vi "VsEP Init Data File.vi"(0 "Expt State":T5, 1 "Params":T2 {"STIMULUS"."dB STEPSIZE" format="%#_3g"; "STIMULUS"."START dB re 1g/ms" step=5}, 7 "Max Jerk (dB re 1 g/ms)":dbl, 11 "error in (no error)":errorcluster) -> (4 "Expt State out":T5, 6 "Datafile path":path, 15 "error out":errorcluster)   [LabVIEW 2020]
uses:
  CFTS Main Panel SubVIs/CFTS-Experiment State.ctl
  Typedefs/VsEP-Parameters.ctl
  Typedefs/VsEP-Stimulus Control.ctl
  Typedefs/VsEP-Hidden Params.ctl
  epl-vi-lib/Signal Synthesis VIs/Controls/Gate XCtl/Gate Control.xctl
  CFTS Main Panel SubVIs/CFTS-Data Type Enum.ctl
  epl-vi-lib/Utility VIs/File IO VIs/Configuration File Wrapper VIs/Config-Read Key (string).vi
panel:
  in  "VsEP Data File":T1
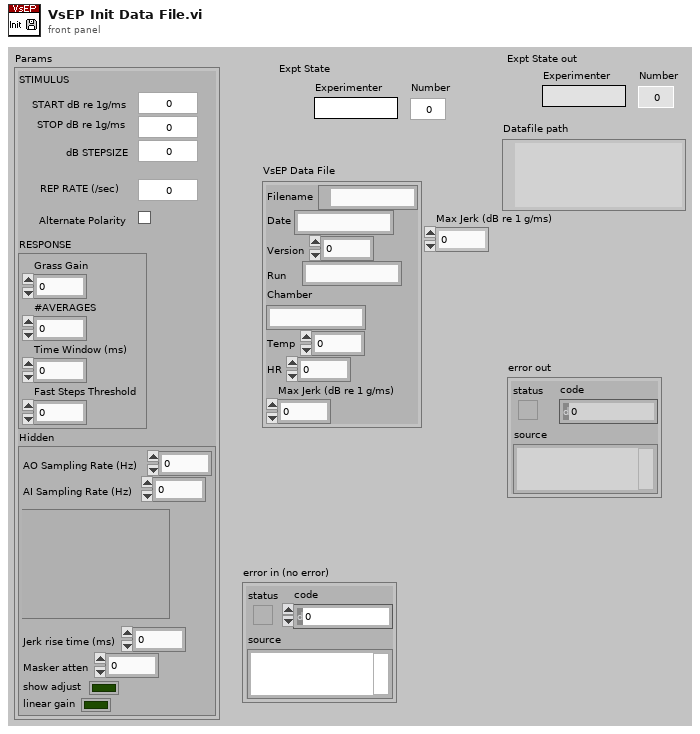
[diagram p1: front panel]
types:
  T1 = cluster{"Filename":path, "Date":string, "Version":i32, "Run":string, "Chamber":string, "Temp":dbl, "HR":dbl, "Max Jerk (dB re 1 g/ms)":dbl}
  T2 = typedef "VsEP-Parameters.ctl" = cluster{"STIMULUS":T3, "RESPONSE":cluster{"Grass Gain":i32, "#AVERAGES":i32, "Time Window (ms)":sgl, "Fast Steps Threshold":i32}, "Hidden":T4}
  T3 = typedef "VsEP-Stimulus Control.ctl" = cluster{"START dB re 1g/ms":i32, "STOP dB re 1g/ms":i32, "dB STEPSIZE":sgl, "REP RATE (/sec)":dbl, "Alternate Polarity":bool, "Sampling Rate (Hz)":dbl}
  T4 = typedef "VsEP-Hidden Params.ctl" = cluster{"AO Sampling Rate (Hz)":dbl, "AI Sampling Rate (Hz)":dbl, "Masker Timing":cluster{"Active":bool, "Delay (ms)":dbl, "Width (ms)":dbl, "Ramp (ms)":dbl}, "Jerk rise time (ms)":dbl, "Masker atten":dbl, "show adjust":bool, "linear gain":bool}
  T5 = typedef "CFTS-Experiment State.ctl" = cluster{"Experimenter":string, "Number":u32, "Right":string, "Left":string, "Data Folder":path, "State File":path, "Version Info":string, "End Exposure Time":dbl, "Exposure Duration":string, "Run #":cluster{"CAP":i16, "ABR":i16, "DP":i16, "VsEP":i16, "MeasSeq":i16, "SubSeq":i16, "SFOAE":i16}}
  T6 = typedef "CFTS-Data Type Enum.ctl" = enum16{"CAP", "ABR", "DP", "VsEP", "MeasSeq", "SFOAE"}
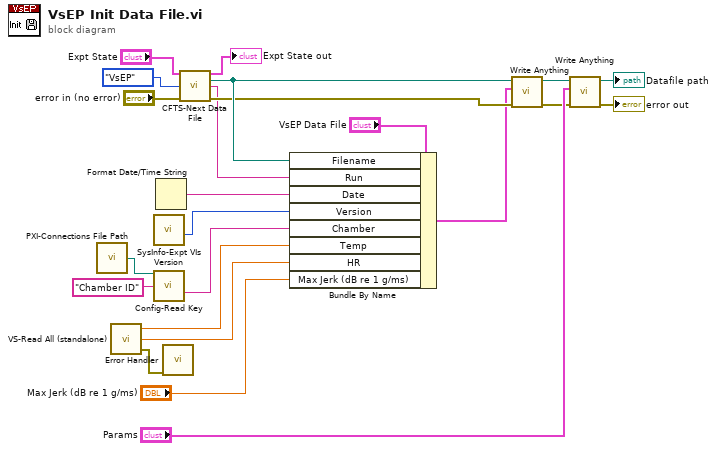
[diagram p0: block diagram]
diagram:
  n1 = call "PXI-Connections File Path.vi"() -> ("Path"=w17:path)  [unwired: 1 in]
  n2 = call "VS-Read All (standalone).vi"() -> ("error out"=w19:errorcluster, "Heart Rate (bpm)"=w3:dbl, "Temperature (C)"=w4:dbl)  [unwired: 3 in]
  n3 = call "SysInfo-Expt VIs Version.vi"() -> ("Expt VIs Version out"=w10:i32)  [unwired: 11 in]
  n4 = call-poly "Config-Read Key.vi"("configuration file path"=w17, "key"="Chamber ID" ("string")) -> ("value"=w5:string)  [unwired: 10 in, 3 out]
  n5 = Format Date/Time String() -> (date/time string=w11:string)  [unwired: 3 in]
  n6 = call "Error Handler.vi"("error in (no error)"=w19) -> ()  [unwired: 13 in, 2 out]
  n7 = call "CFTS-Next Data File.vi"("Expt State"="Expt State", "Data Type"=CFTS-Data_Type_Enum."VsEP", "error in (no error)"="error in (no error)") -> ("Expt State out"=→"Expt State out":T5, "Datafile path"=w9:path, "run #"=w1:string, "error out"=w7:errorcluster)  [unwired: 8 in, 1 out]
  n8 = Bundle By Name(cluster="VsEP Data File", "Filename"=w9, "Run"=w1, "Date"=w11, "Version"=w10, "Chamber"=w5, "Temp"=w4, "HR"=w3, "Max Jerk (dB re 1 g/ms)"="Max Jerk (dB re 1 g/ms)") -> (w6:T1)
  n9 = call "Write Anything.vi"("Error In"=w7, "Anything"=w6, "Path (dialog)"=w9) -> ("Error Out"=w13:errorcluster, "Path out"=w14:path)  [unwired: 7 in]
  n10 = call "Write Anything.vi"("Error In"=w13, "Anything"="Params", "Path (dialog)"=w14) -> ("Error Out"=→"error out":errorcluster, "Path out"=→"Datafile path":path)  [unwired: 7 in]
